vi "Generate Start-Up Registry Patch File.vi"(6 "registry path":T1(ring), 7 "RegPath":path, 8 "error in (no error)":errorcluster, 9 "Key Name(Empty to use exe name)":string, 10 "Arguments":string, 11 "EXE Path":path) -> (0 "error out":errorcluster)   [LabVIEW 2020]
panel:
  out "resulting string":string
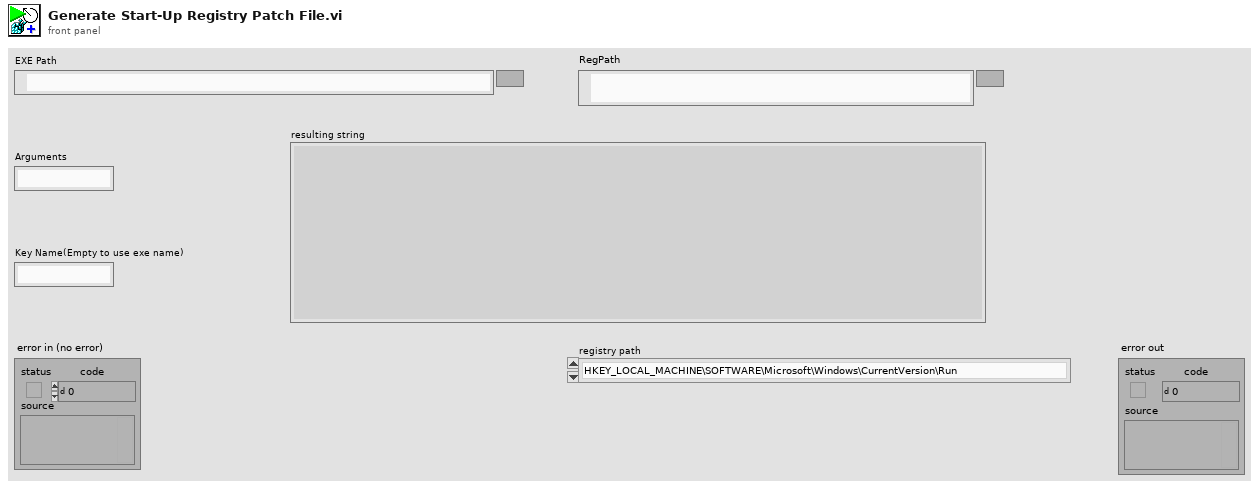
[diagram p1: front panel]
types:
  T1 = enum16{"HKEY_LOCAL_MACHINE\\SOFTWARE\\Microsoft\\Windows\\CurrentVersion\\Run", "HKEY_LOCAL_MACHINE\\Software\\Microsoft\\Windows\\CurrentVersion\\RunOnce", "HKEY_CURRENT_USER\\Software\\Microsoft\\Windows\\CurrentVersion\\Run", "HKEY_CURRENT_USER\\Software\\Microsoft\\Windows\\CurrentVersion\\RunOnce"}
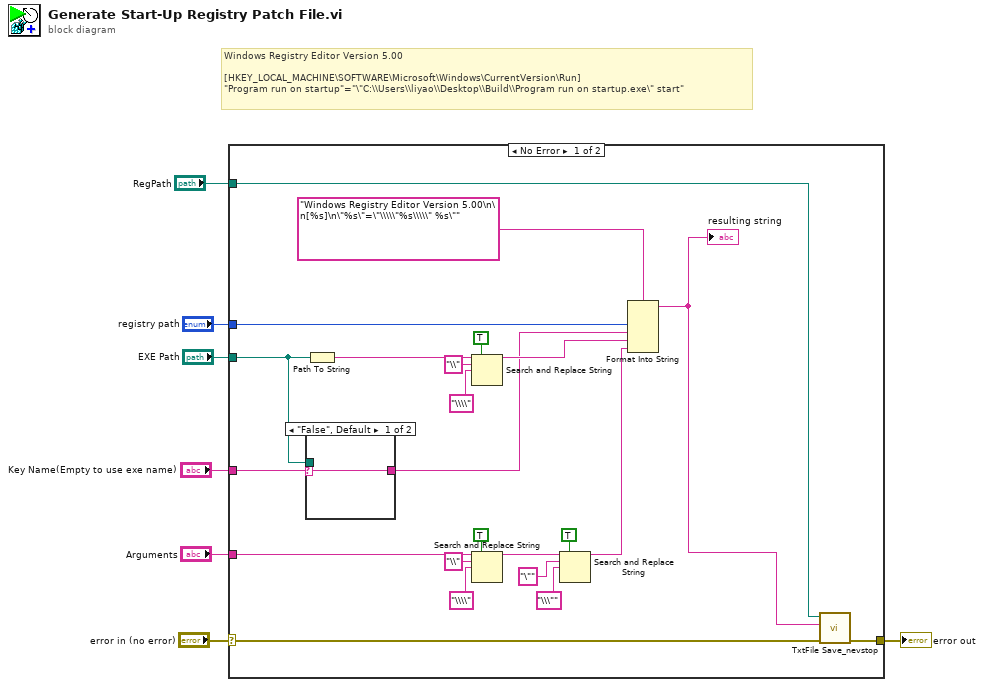
[diagram p0: block diagram]
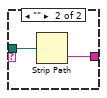
[diagram p2: hidden frame]
diagram:
  # "Windows Registry Editor Version 5.00\n\n[HKEY_LOCAL_MACHINE\\SOFTWARE\\Microsoft\\Windows\\CurrentVersion\\Run]\n\"Program run on startup\"=\"\\\"C:\\\\Users\\\\liyao\\\\Desktop\\\\Build\\\\Program run on startup.exe\\\" start\""
  n1 = case shown="No Error" "error in (no error)" {
    selector: "error in (no error)" -> [w11 w34]
    tunnel: "registry path" -> [w30 _]
    tunnel: "EXE Path" -> [w29 _]
    tunnel: "Key Name(Empty to use exe name)" -> [w24 _]
    tunnel: "Arguments" -> [w20 _]
    tunnel: [w10 w34] -> w2
    tunnel: "RegPath" -> [w8 _]
    frame No Error {
      n2 = case shown="\"False\", Default" w24 {
        selector: w24 -> [w31 _]
        tunnel: w29 -> [_ w33]
        tunnel: [w31 w32] -> w12
        frame "False", Default {
        }
        frame "" {
          n3 = Strip Path(path=w33) -> (name=w32:string)  [unwired: 1 out]
        }
      }
      n4 = Path To String(path=w29) -> (string=w28:string)
      n5 = Search and Replace String(replace all?=TRUE ("replace all? (F)"), input string=w28, search string="\\", replace string="\\\\" ("search string")) -> (result string=w13:string)  [unwired: 4 in, 3 out]
      n6 = Search and Replace String(replace all?=TRUE ("replace all? (F)"), input string=w20, search string="\\", replace string="\\\\" ("search string")) -> (result string=w16:string)  [unwired: 4 in, 3 out]
      n7 = Search and Replace String(replace all?=TRUE ("replace all? (F)"), input string=w16, search string="\"", replace string="\\\"" ("search string")) -> (result string=w14:string)  [unwired: 4 in, 3 out]
      n8 = Format Into String(format string="Windows Registry Editor Version 5.00\n\n[%s]\n\"%s\"=\"\\\\\"%s\\\\\" %s\"", w30, w12, w13, w14) -> (resulting string=w9:string)  [unwired: 2 in, 1 out]
      "resulting string" <- w9
      n9 = call <userlib>:"TxtFile Save_nevstop.vi"("error in (no error)"=w11, "text"=w9, "Path"=w8) -> ("error out"=w10:errorcluster)  [unwired: 8 in]
    }
    frame Error {
    }
  }
  "error out" <- w2
